vi "Translate Data.vi"(8 "error in (no error)":errorcluster, 10 "DataBuffer":string, 11 "Alicat_VC in":refnum<class "Alicat_VC.lvclass">) -> (0 "error out":errorcluster, 2 "DataOut":refnum<class "Data.lvclass">, 3 "Alicat_VC out":refnum<class "Alicat_VC.lvclass">)   [LabVIEW 2014, in "Alicat.lvlib" / "Alicat_VC.lvclass"]
doc: "VI used to translate the data buffer to something meaningful (implementation dependent). This VI must be overridden."
uses:
  Alicat_VC.lvclass
  reusable/Data/Data.lvclass
  Data/VC/AlicatVCData.lvclass
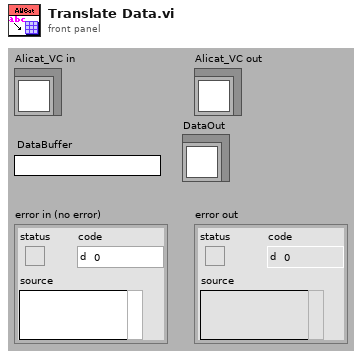
[diagram p1: front panel]
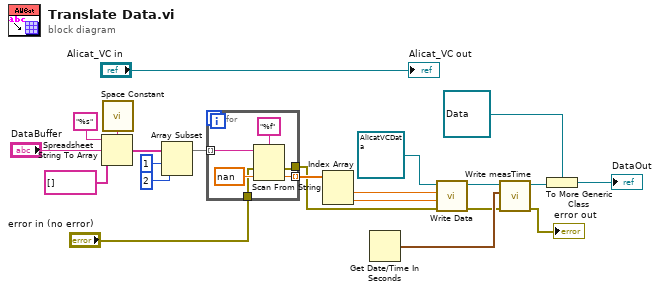
[diagram p0: block diagram]
diagram:
  n1 = call <vilib>:"Space Constant.vi"() -> ("String"=w21:string)
  n2 = Spreadsheet String To Array(delimiter (Tab)=w21, format string="%s", spreadsheet string="DataBuffer", array type (2D Dbl)=string[] []) -> (array=w7:string[])
  n3 = Array Subset(array=w7, index=1, length=2) -> (w4:string[])
  n4 = for {
    tunnel: w4 -> [w28] mode=indexing
    tunnel: [w25] -> w16 mode=indexing
    tunnel: "error in (no error)" -> [w24]
    tunnel: [w23] -> w9
    n5 = Scan From String(format string="%f", input string=w28, error in=w24, default 1=sgl nan ("default value 1")) -> (error out=w23:errorcluster, output 1=w25:sgl)  [unwired: 1 in, 2 out]
  }
  n6 = Index Array(array=w16) -> (element #1=w15:sgl, element #2=w14:sgl)  [unwired: 2 in]
  n7 = Get Date/Time In Seconds() -> (seconds since 1Jan1904=w12:timestamp)
  n8 = call "Write Data.vi"("error in (no error)"=w9, "Qsp"=w14, "Q"=w15, "AlicatVData in"=refnum<class "AlicatVCData.lvclass"> refnum) -> ("error out"=w11:errorcluster, "AlicatVData out"=w13:refnum<class "AlicatVCData.lvclass">)  [unwired: 6 in]
  n9 = call "Write measTime.vi"("error in (no error)"=w11, "measTime"=w12, "Data in"=w13) -> ("error out"=→"error out":errorcluster, "Data out"=w3:refnum<class "AlicatVCData.lvclass">)  [unwired: 7 in]
  n10 = To More Generic Class(target class=refnum<class "Data.lvclass"> refnum ("DataOut"), reference=w3) -> (generic class reference=→"DataOut":refnum<class "Data.lvclass">)
  "Alicat_VC out" <- "Alicat_VC in"
